vi "删除数据到配置文件段.vi"(8 "错误输入（无错误）":errorcluster, 9 "refnum":T1, 11 "Ring输入":refnum<vi>) -> (0 "错误输出":errorcluster, 3 "引用句柄输出":T1 caption="refnum out")   [LabVIEW 2015]
uses:
  <vilib>/Utility/config.llb/Config Data RefNum.ctl
  <vilib>/Utility/config.llb/NI_LVConfig.lvlib
panel:
  out "已删除的部分":string
  out "section exists?":bool caption="段存在？"
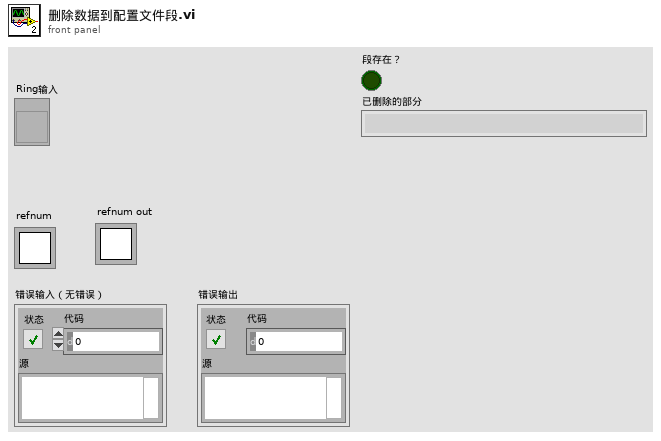
[diagram p1: front panel]
types:
  T1 = typedef "NI_LVConfig.lvlib/Config Data RefNum.ctl" = refnum<k1>
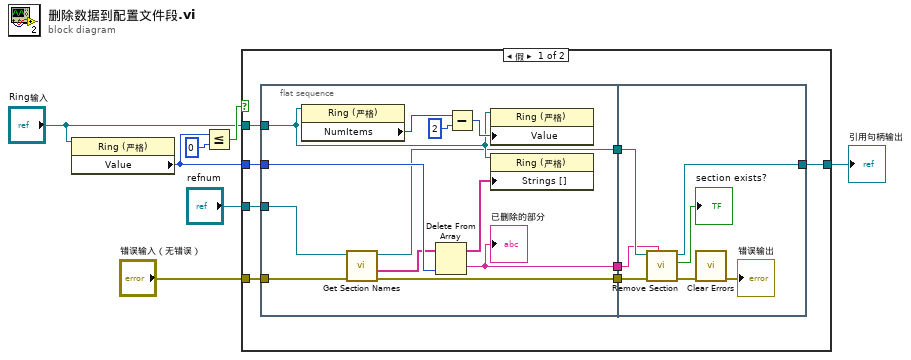
[diagram p0: block diagram]
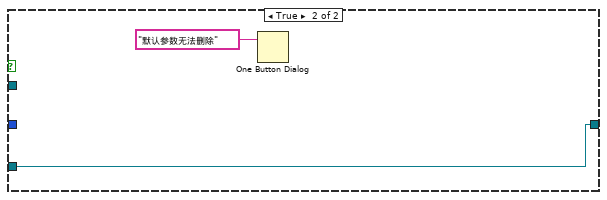
[diagram p2: hidden frame]
diagram:
  n1 = property on="属性节点" class="Ring (严格)"(reference="Ring输入") -> ("Value"=w5:u16)  [unwired: 1 in, 2 out]
  n2 = Less Or Equal?(x=w5, y=u16 0) -> (x <= y?=w7:bool)
  n3 = case shown="假" w7 {
    tunnel: w5 -> [w15 _]
    tunnel: "Ring输入" -> [w14 _]
    tunnel: "refnum" -> [w11 w35]
    tunnel: [w12 w35] -> w2
    tunnel: "错误输入（无错误）" -> [w10 _]
    frame False {
      n4 = flat-sequence {
        tunnel: w15 -> [w26]
        tunnel: w14 -> [w22]
        tunnel: [w21] -> w13
        tunnel: w11 -> [w20]
        tunnel: w10 -> [w19]
        tunnel: [w17] -> w9
        tunnel: [w16] -> w8
        tunnel: w13 -> [w28]
        tunnel: [w31] -> w12
        tunnel: w9 -> [w30]
        tunnel: w8 -> [w29]
        frame #0 {
          n5 = property on="属性节点" class="Ring (严格)"(reference=w22) -> ("NumItems"=w24:u32)  [unwired: 1 in, 2 out]
          n6 = call <vilib>:"Get Section Names.vi"("error in (no error)"=w19, "refnum"=w20) -> ("error out"=w17:errorcluster, "section names"=w18:string[], "refnum out"=w16:T1)  [unwired: 7 in]
          n7 = Delete From Array(array=w18, index=w26) -> (deleted portion=w21:string, array with subset deleted=w27:string[])  [unwired: 1 in]
          "已删除的部分" <- w21
          n8 = Subtract(x=w24, y=u32 2) -> (x-y=w25:u32)
          n9 = property on="属性节点" class="Ring (严格)"(reference=w22, "Value"=w25) -> ()  [unwired: 1 in, 2 out]
          n10 = property on="属性节点" class="Ring (严格)"(reference=w22, "Strings []"=w27) -> ()  [unwired: 1 in, 2 out]
        }
        frame #1 {
          n11 = call <vilib>:"Remove Section.vi"("section"=w28, "error in (no error)"=w30, "refnum"=w29) -> ("error out"=w33:errorcluster, "section exists?"=→"section exists?":bool, "refnum out"=w31:T1)  [unwired: 6 in]
          n12 = call <vilib>:"Clear Errors.vi"("error in (no error)"=w33) -> ("error out"=→"错误输出":errorcluster)  [unwired: 5 in, 1 out]
        }
      }
    }
    frame True {
      n13 = One Button Dialog(message="默认参数无法删除" ("消息")) -> ()  [unwired: 1 in, 1 out]
    }
  }
  "引用句柄输出" <- w2
